vi "reshapeArray.vi"(7 "reshapeInfo":T2, 9 "element":T1, 10 "center":i32, 11 "z":dbl[][](array[numeric])) -> (3 "reshaped array":dbl[](array[numeric]))   [LabVIEW 2011]
uses:
  reshapeINfo_TypDef.ctl
  emptyArray_TYpDEf.ctl
  emptyArrayCamX_TypDef.ctl
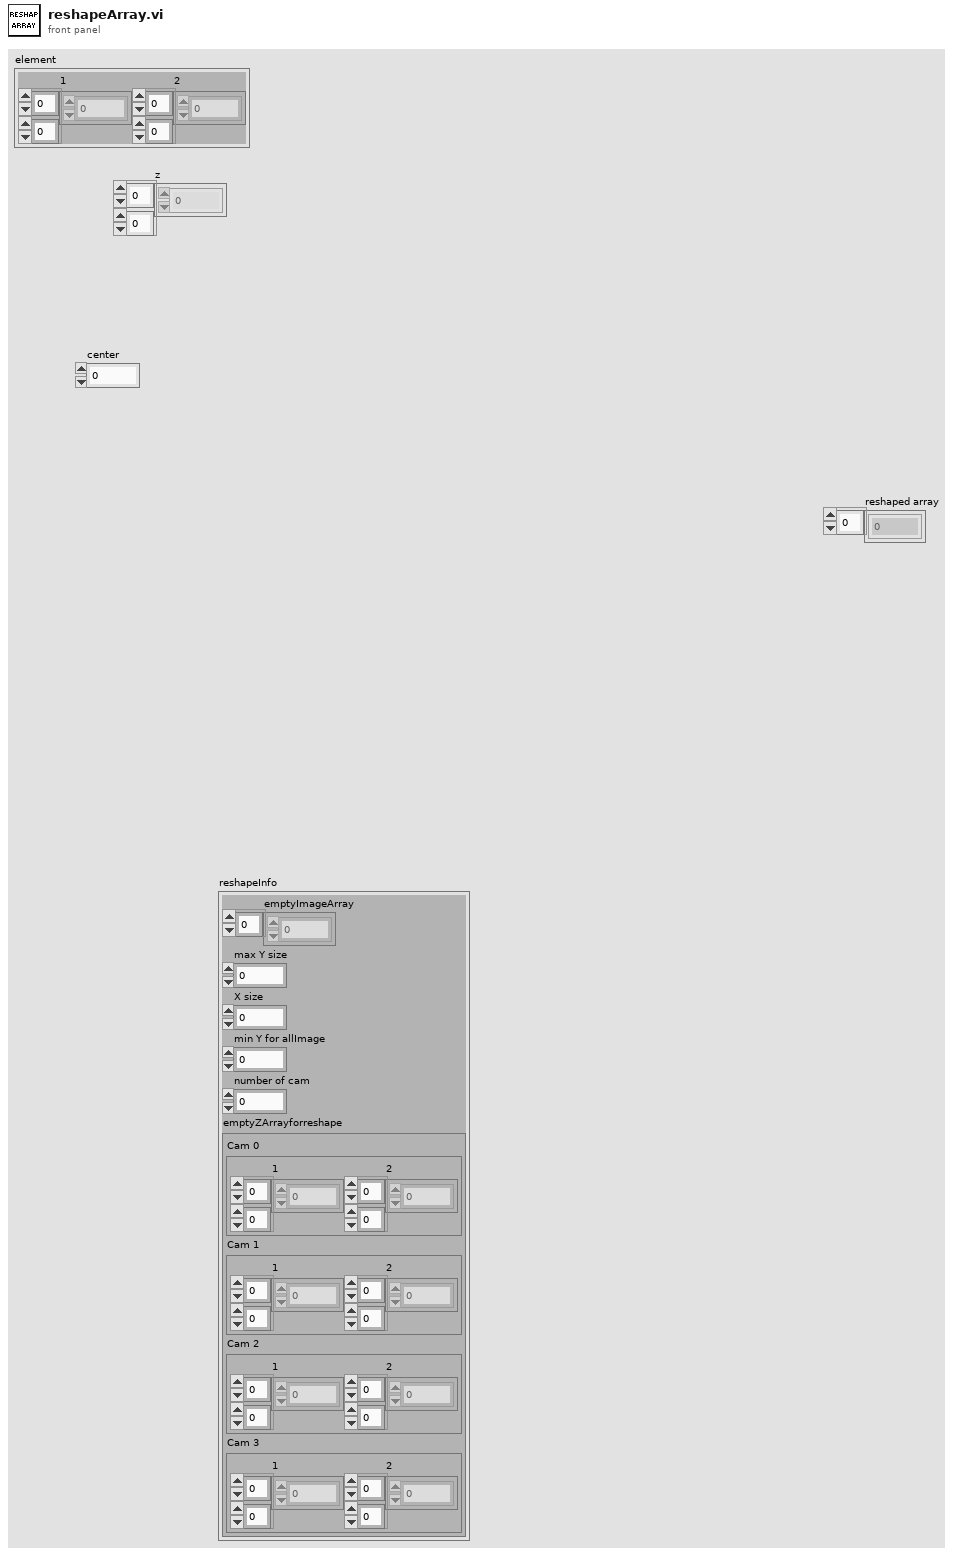
[diagram p1: front panel]
types:
  T1 = typedef "emptyArrayCamX_TypDef.ctl" = cluster{"1":dbl[][], "2":dbl[][]}
  T2 = typedef "reshapeINfo_TypDef.ctl" = cluster{"emptyImageArray":dbl[], "max Y size":i32, "X size":i32, "min Y for allImage":dbl, "number of cam":i32, "emptyZArrayforreshape":T3}
  T3 = typedef "emptyArray_TYpDEf.ctl" = cluster{"Cam 0":T1, "Cam 1":T1, "Cam 2":T1, "Cam 3":T1}
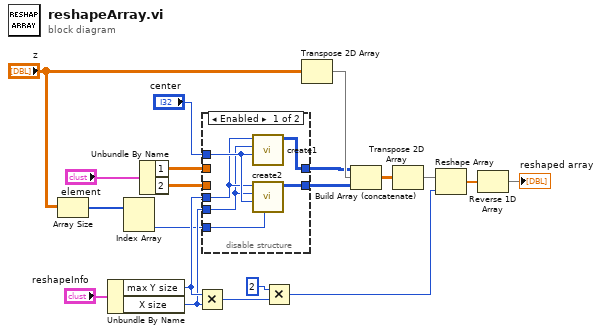
[diagram p0: block diagram]
diagram:
  n1 = Array Size(array="z") -> (size(s)=w1:i32[])
  n2 = Unbundle By Name("reshapeInfo") -> ("max Y size"=w15:i32, "X size"=w14:i32)
  n3 = Index Array(array=w1) -> (element #2=w7:i32)  [unwired: 2 in, 1 out]
  n4 = Unbundle By Name("element") -> ("1"=w6:dbl[][], "2"=w5:dbl[][])
  n5 = Multiply(x=w15, y=w14) -> (x*y=w13:i32)
  n6 = disable-structure shown="Enabled" {
    disable-tunnel: "center" -> [w26 _]
    disable-tunnel: [w25 w28] -> w3
    disable-tunnel: [w24 w27] -> w2
    disable-tunnel: w15 -> [w23 _]
    disable-tunnel: w14 -> [w22 _]
    disable-tunnel: w7 -> [w21 _]
    disable-tunnel: w6 -> [_ w28]
    disable-tunnel: w5 -> [_ w27]
    frame Enabled {
      n7 = call "create1.vi"("center"=w26, "X size"=w22, "max Y size"=w23) -> ("Array"=w25:i32[][])  [unwired: 7 in, 1 out]
      n8 = call "create2.vi"("actual y size"=w21, "center"=w26, "X size"=w22, "max Y size"=w23) -> ("Array"=w24:i32[][])  [unwired: 6 in, 1 out]
    }
    frame Disabled {
    }
  }
  n9 = Multiply(x=2, y=w13) -> (x*y=w11:i32)
  n10 = Transpose 2D Array(2D array="z") -> (transposed array=w9:dbl[][])
  n11 = Build Array (concatenate)(w3, w9, w2) -> (w10:dbl[][])
  n12 = Transpose 2D Array(2D array=w10) -> (transposed array=w17:dbl[][])
  n13 = Reshape Array(w17, w11) -> (w16:dbl[])
  n14 = Reverse 1D Array(array=w16) -> (reversed array=→"reshaped array":dbl[])
